vi "compute rates_fixed.vi"(0 "Host Plot Controls":T1={"refresh"=FALSE, "PMTs for Host"={"Sa"=0, "Sb"=1, "g-factor"=1}, "Peaks"={"# bins"=1000, "min"=0.020751953125, "max"=0.00103759765625}, "Averages"={"# bins"=1000, "max"=0.020751953125, "min"=0.00103759765625}, "Durations"={"# bins"=1000, "max"=20.0, "min"=8.0}, "FP-FPGA"={"# bins"=1000, "max"=20.0, "min"=8.0}, "FP-Host"={"# bins"=1000, "max"=20.0, "min"=8.0}, "Max or Average"=0} {"Max or Average" items=["Peak Max", "Peak Average"]}, 7 "peaks data":T4, 12 "shifts in":T2) -> (2 "dropfreq":dbl, 3 "sortfreq":dbl, 4 "number detected":i32, 6 "number sorted":i32, 14 "shifts out":T3, 15 "number drops just detected":i32)   [LabVIEW 2009]
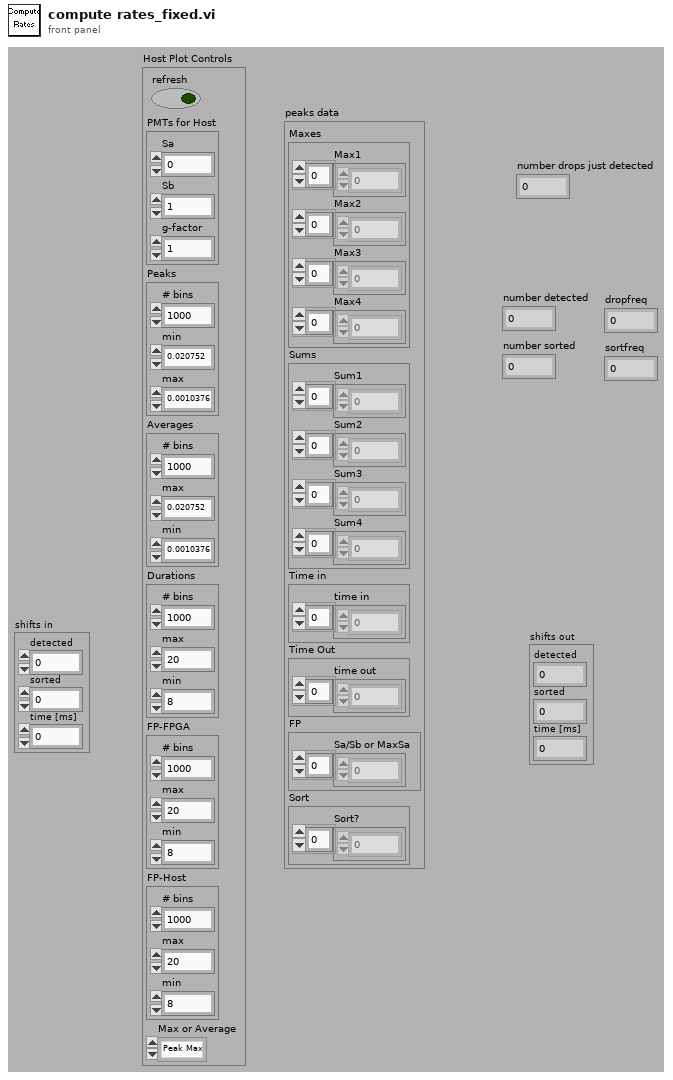
[diagram p1: front panel]
types:
  T1 = cluster{"refresh":bool, "PMTs for Host":cluster{"Sa":i8, "Sb":i8, "g-factor":i32}, "Peaks":cluster{"# bins":i32, "min":dbl, "max":dbl}, "Averages":cluster{"# bins":i32, "max":dbl, "min":dbl}, "Durations":cluster{"# bins":i32, "max":dbl, "min":dbl}, "FP-FPGA":cluster{"# bins":i32, "max":dbl, "min":dbl}, "FP-Host":cluster{"# bins":i32, "max":dbl, "min":dbl}, "Max or Average":i8}
  T2 = cluster{"detected":i32, "sorted":i32, "time [ms]":u32}
  T3 = cluster{"detected":i32, "sorted":dbl, "time [ms]":u32}
  T4 = cluster{"Maxes":cluster{"Max1":dbl[], "Max2":dbl[], "Max3":dbl[], "Max4":dbl[]}, "Sums":cluster{"Sum1":dbl[], "Sum2":dbl[], "Sum3":dbl[], "Sum4":dbl[]}, "Time in":cluster{"time in":dbl[]}, "Time Out":cluster{"time out":dbl[]}, "FP":cluster{"Sa/Sb or MaxSa":dbl[]}, "Sort":cluster{"Sort?":dbl[]}}
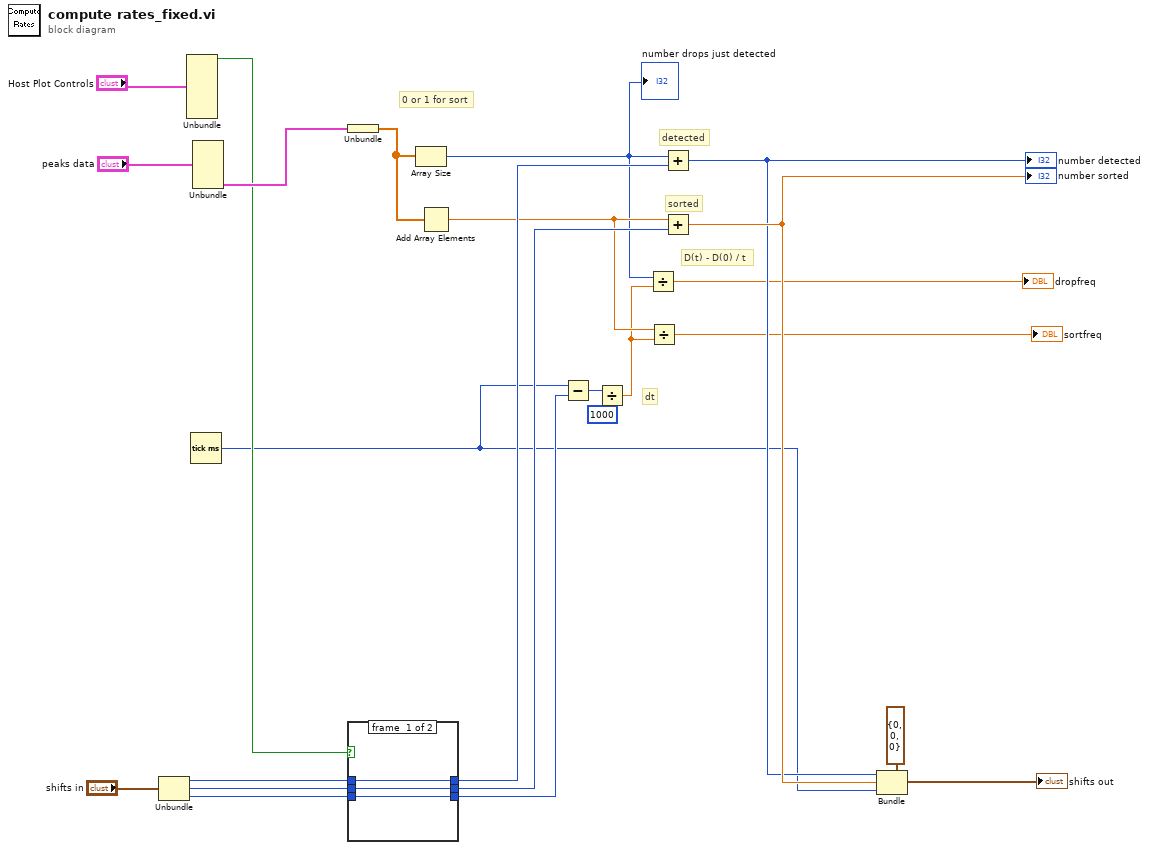
[diagram p0: block diagram]
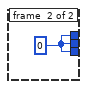
[diagram p2: hidden frame]
diagram:
  # "detected"
  # "sorted"
  # "dt"
  # "D(t) - D(0) / t"
  # "0 or 1 for sort"
  n1 = Unbundle("shifts in") -> ("detected"=w17:i32, "sorted"=w16:i32, "time [ms]"=w15:u32)
  n2 = Unbundle("Host Plot Controls") -> ("refresh"=w11:bool)  [unwired: 7 out]
  n3 = Tick Count (ms)() -> (millisecond timer value=w5:u32)
  n4 = Unbundle("peaks data") -> ("Sort"=w23:cluster{"Sort?":dbl[]})  [unwired: 5 out]
  n5 = Unbundle(w23) -> ("Sort?"=w22:dbl[])
  n6 = case shown="True" w11 {
    tunnel: w17 -> [w27 _]
    tunnel: w16 -> [w26 _]
    tunnel: w15 -> [w25 _]
    tunnel: [w27 w28] -> w14
    tunnel: [w26 w28] -> w13
    tunnel: [w25 w28] -> w12
    frame #0 {
    }
    frame #1 {
      w28 = 0
    }
  }
  n7 = Array Size(array=w22) -> (size(s)=w8:i32)
  "number drops just detected" <- w8
  n8 = Add Array Elements(numeric array=w22) -> (sum=w9:dbl)
  n9 = Subtract(x=w5, y=w12) -> (x-y=w4:u32)
  n10 = Divide(x=w4, y=1000) -> (x/y=w2:dbl)
  n11 = Divide(x=w8, y=w2) -> (x/y=→"dropfreq":dbl)
  n12 = Divide(x=w9, y=w2) -> (x/y=→"sortfreq":dbl)
  n13 = Add(x=w8, y=w14) -> (x+y=w10:i32)
  "number detected" <- w10
  n14 = Add(x=w9, y=w13) -> (x+y=w18:dbl)
  "number sorted" <- w18
  n15 = Bundle(cluster=T2 {"detected"=0, "sorted"=0, "time [ms]"=0} ("output cluster"), "detected"=w10, "sorted"=w18, "time [ms]"=w5) -> (→"shifts out":T2)
